vi "Resize.vi"(4 "Send events? [T]":bool=TRUE, 6 "Defer Panel Updates? [T]":bool=TRUE, 7 "VI Refnum":refnum<vi>, 8 "error in (no error)":errorcluster, 10 "Bounds":T1, 11 "MMI Scaling in":refnum<class "IContainer.lvclass">) -> (0 "error out":errorcluster, 2 "Resized":string[](array[string]), 3 "MMI Scaling out":refnum<class "IContainer.lvclass">)   [LabVIEW 2013, in "IContainer.lvclass"]
doc: "Copyright 2018, Wiebe Walstra, wiebe@carya.nl."
uses:
  IContainer.lvclass
  <vilib>/Utility/miscctls.llb/LVRectTypeDef.ctl
  IObject.lvclass
  IContainer.lvclass/IContainer.ctl
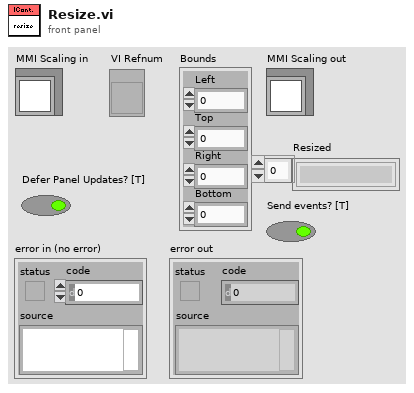
[diagram p1: front panel]
types:
  T1 = typedef "LVRectTypeDef.ctl" = cluster{"Left":i16, "Top":i16, "Right":i16, "Bottom":i16}
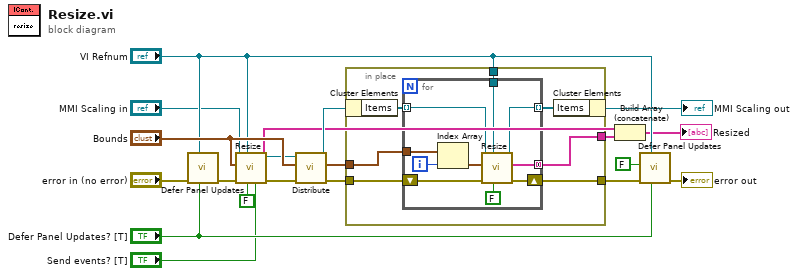
[diagram p0: block diagram]
diagram:
  n1 = call "Defer Panel Updates.vi"("Set Defer Panel Updates? [T]"="Defer Panel Updates? [T]", "VI Refnum"="VI Refnum", "error in (no error)"="error in (no error)") -> ("error out"=w1:errorcluster)  [unwired: 8 in]
  n2 = call-parent "Resize.vi"("Send events? [T]"="Send events? [T]", "Defer Panel Updates? [T]"=FALSE, "VI Refnum"="VI Refnum", "error in (no error)"=w1, "Bounds"="Bounds", "MMI Scaling in"="MMI Scaling in") -> ("error out"=w3:errorcluster, "Resized"=w6:string[], "MMI Scaling out"=w9:refnum<class "IContainer.lvclass">)  [unwired: 3 in]
  n3 = call-dynamic "Distribute.vi"("error in (no error)"=w3, "Bounds"="Bounds", "Container in"=w9) -> ("error out"=w17:errorcluster, "Bounds"=w15:T1[], "Container out"=w16:refnum<class "IContainer.lvclass">)  [unwired: 4 in, 2 out]
  n4 = in-place {
    in-place-border: [w26] -> w18
    in-place-border: w17 -> [w25]
    in-place-border: w15 -> [w22]
    in-place-border: "VI Refnum" -> [w24]
    in-place-border: [w21] -> w11
    n5 = in-place-cluster #1(w16) -> ("Items"=w23:refnum<class "IObject.lvclass">[])
    n6 = for {
      tunnel: [w35] -> w27 mode=indexing
      tunnel: w23 -> [w28] mode=indexing
      shift-right: [w36] -> w26
      shift-left: w25 -> [w37]
      tunnel: w22 -> [w32]
      tunnel: w24 -> [w34]
      tunnel: [w29] -> w21 mode=concatenating
      i -> [w31]
      n7 = Index Array(array=w32, index=w31) -> (element=w30:T1)
      n8 = call-dynamic "Resize.vi"("Defer Panel Updates? [T]"=FALSE, "VI Refnum"=w34, "error in (no error)"=w37, "Bounds"=w30, "MMI Scaling in"=w28) -> ("error out"=w36:errorcluster, "Resized"=w29:string[], "MMI Scaling out"=w35:refnum<class "IObject.lvclass">)  [unwired: 4 in]
    }
    n9 = in-place-cluster #1("Items"=w27) -> (→"MMI Scaling out":refnum<class "IContainer.lvclass">)
  }
  n10 = Build Array (concatenate)(w6, w11) -> (→"Resized":string[])
  n11 = call "Defer Panel Updates.vi"("Set Defer Panel Updates? [T]"="Defer Panel Updates? [T]", "VI Refnum"="VI Refnum", "error in (no error)"=w18, "Defer Panel Updates? [T]"=FALSE) -> ("error out"=→"error out":errorcluster)  [unwired: 7 in]
